vi "Get Sentence Type.vi"(8 "error in (no error)":errorcluster, 11 "sentence":string) -> (0 "error out":errorcluster, 1 "valid sentence?":bool, 3 "sentence type":string)   [LabVIEW 2024]
uses:
  <vilib>/regexp/Match Regular Expression.xnode
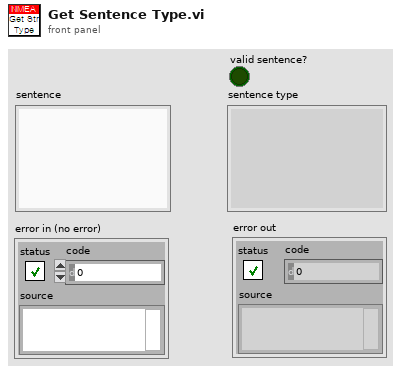
[diagram p1: front panel]
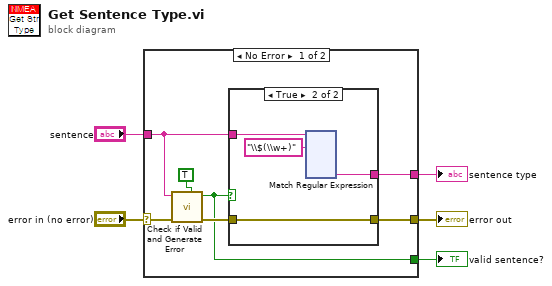
[diagram p0: block diagram]
diagram:
  n1 = case shown="No Error" "error in (no error)" {
    selector: "error in (no error)" -> [w10 w137]
    tunnel: [w11 w137] -> w5
    tunnel: [w12 _] -> w4
    tunnel: "sentence" -> [w8 _]
    tunnel: [w7 _] -> w1
    frame No Error {
      n2 = call "Check if Valid and Generate Error.vi"("generate error if invalid (F)"=TRUE, "error in (no error)"=w10, "sentence"=w8) -> ("error out"=w9:errorcluster, "valid sentence"=w7:bool)  [unwired: 7 in]
      n3 = case shown="True" w7 {
        tunnel: [_ w16] -> w12
        tunnel: [w13 w15] -> w11
        tunnel: w9 -> [w13 w15]
        tunnel: w8 -> [_ w14]
        frame False {
          # "Invalid sentence"
        }
        frame True {
          n4 = xnode "Match Regular Expression"("입력 문자열"=w14, "정규식"="\\$(\\w+)" ("regular expression")) -> ("부분 일치 1"=w16:string)  [unwired: 2 in, 7 out]
        }
      }
    }
    frame Error {
      # "If there is an error coming in,\nthen it just returns that error\nand an empty string"
    }
  }
  "sentence type" <- w4
  "error out" <- w5
  "valid sentence?" <- w1
